vi "subStage_Calibrate.vi"(6 "Stage Info":T1={" Current Position"=[-1.0, -12.0, 0.0], "Number of Axis"=3, "ILSID"=1}, 7 "error in (no error)":errorcluster) -> (0 "error out":errorcluster, 4 "Calibrate":bool)   [LabVIEW 2015]
panel:
  # "X"
  # "Y"
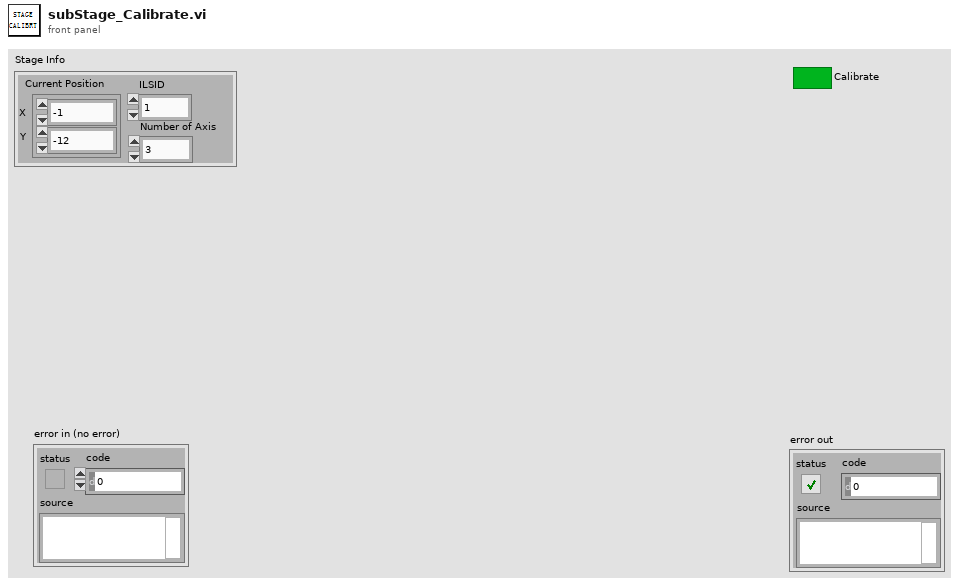
[diagram p1: front panel]
types:
  T1 = cluster{" Current Position":dbl[], "Number of Axis":i32, "ILSID":i32}
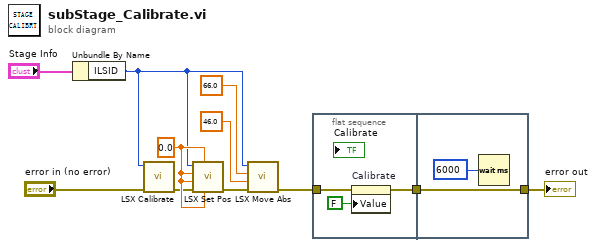
[diagram p0: block diagram]
diagram:
  w10 = 0.0 ("dX")
  n1 = Unbundle By Name("Stage Info") -> ("ILSID"=w3:i32)
  n2 = call <userlib>:"LSX Calibrate.vi"("error in (no error)"="error in (no error)", "lLSID"=w3) -> ("error out"=w9:errorcluster)  [unwired: 8 in, 1 out]
  n3 = call <userlib>:"LSX Set Pos.vi"("dA"=w10, "dZ"=w10, "error in (no error)"=w9, "dY"=w10, "dX"=w10, "lLSID"=w3) -> ("error out"=w8:errorcluster)  [unwired: 4 in, 1 out]
  n4 = call <userlib>:"LSX Move Abs.vi"("error in (no error)"=w8, "dY"=46.0, "dX"=66.0, "lLSID"=w3) -> ("error out"=w11:errorcluster)  [unwired: 6 in, 1 out]
  n5 = flat-sequence {
    tunnel: w11 -> [w14]
    tunnel: [w13] -> w1
    tunnel: [w15] -> w5
    tunnel: w1 -> [w15]
    frame #0 {
      n6 = property on="Calibrate" class="Bool (strict)"(error in=w14, "Value"=FALSE ("Calibrate")) -> (error out=w13:errorcluster)  [unwired: 1 in, 1 out]
    }
    frame #1 {
      n7 = Wait (ms)(milliseconds to wait=u32 6000) -> ()  [unwired: 1 out]
    }
  }
  "error out" <- w5
